vi "Destroy.vi"(8 "error in (no error)":errorcluster, 11 "reference in":refnum<class "Camera_IMAQdx.lvclass">) -> (0 "error out":errorcluster, 3 "reference out":refnum<class "Camera_IMAQdx.lvclass">)   [LabVIEW 2017, in "Camera_IMAQdx.lvclass"]
uses:
  Camera_IMAQdx.lvclass
  Camera_class/Camera.lvclass
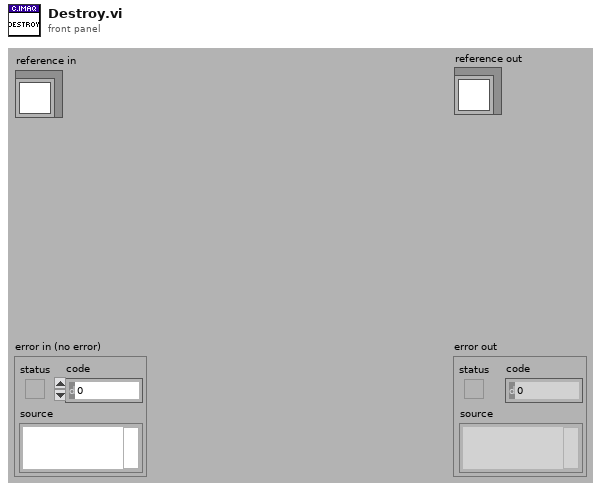
[diagram p1: front panel]
types:
  T1 = typedef "Camera_IMAQdx.lvclass/ObjectAttributes.ctl" = cluster{"Configuration":T2, "Session":T3, "Connected":bool, "Image":T4, "Grab Frame Number":u32}
  T2 = typedef "Camera_IMAQdx.lvclass/Configuration--Cluster.ctl" = cluster{"Camera Interface Name":string, "Number of Buffers":u32, "Image Name":string}
  T3 = typedef "IMAQdx.ctl" = refnum<k21>
  T4 = typedef "IMAQ Image.ctl" = refnum<image>
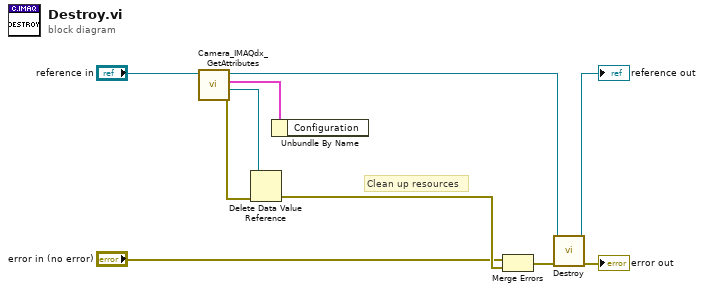
[diagram p0: block diagram]
diagram:
  # "Clean up resources"
  n1 = call "Camera_IMAQdx_GetAttributes.vi"("reference in"="reference in") -> ("error out"=w9:errorcluster, "DataRef"=w8:refnum<data-value>, "Data"=w7:T1, "reference out"=w4:refnum<class "Camera_IMAQdx.lvclass">)  [unwired: 7 in]
  n2 = Delete Data Value Reference(data value reference=w8, error in=w9) -> (error out=w6:errorcluster)  [unwired: 1 out]
  n3 = Unbundle By Name(w7) -> ()  [unwired: 1 out]
  n4 = Merge Errors("error in (no error)", w6) -> (w2:errorcluster)
  n5 = call-parent "Destroy.vi"("error in (no error)"=w2, "reference in"=w4) -> ("error out"=→"error out":errorcluster, "reference out"=→"reference out":refnum<class "Camera_IMAQdx.lvclass">)  [unwired: 8 in]
